vi "scanpic.vi"(8 "error in (no error)":errorcluster, 9 "Size (m)":cluster{"Width":sgl, "Height":sgl}={"Width"=nan, "Height"=nan} caption="Size (m) (NaN=no change)" {"Height" format="%.2p"; "Width" format="%.2p"}, 10 "Application ref in":refnum<vi>, 11 "Center coordinates (m)":cluster{"Xc":sgl, "Yc":sgl}={"Xc"=nan, "Yc"=nan} caption="Center coordinates (m) (NaN=no change)" {"Yc" format="%.2p"; "Xc" format="%.2p"}) -> (0 "Error out":errorcluster, 2 "Application ref out":refnum<vi>, 3 "Data":sgl[][](array[numeric]) format="%#_5p")   [LabVIEW 2020]
uses:
  <userlib>/Nanonis Prog Interface V5/Nanonis Prog Interface.lvlib
panel:
  in  "Channels indexes (0-23) 2":i32[](array[numeric]) caption="Channels indexes (0-23) (Empty=no change)"
  out "Channel name":string
  in  "Channel index (0-23)":u8=14
  out "Signals Names":string[](array[string])
  in  "Pixels":i32 caption="Pixels/line (0=no change)"
  out "Lines":i32
  out "Pixels/line":i32
  out "Channels indexes (0-23)":i32[](array[numeric])
  in  "Serie name":string="ScanMultiBias_"
  in  "Bias increment":sgl
  out "Bias voltage":sgl caption="Current bias voltage"
  out "Scan":u8 caption="Current scan"
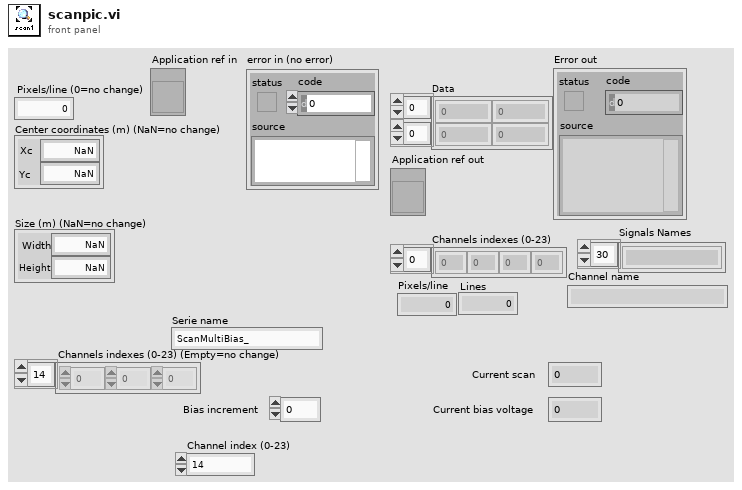
[diagram p1: front panel]
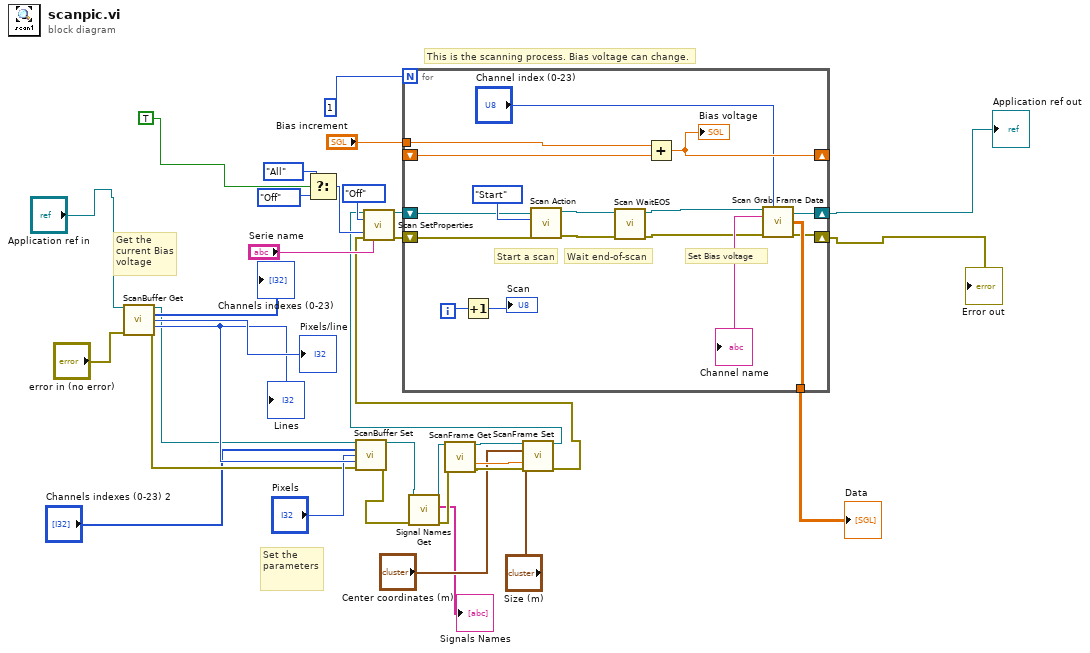
[diagram p0: block diagram]
diagram:
  # "Set the parameters"
  # "This is the scanning process. Bias voltage can change."
  # "Get the current Bias voltage"
  n1 = call <userlib>:"ScanBuffer Get.vi"("Application ref in"="Application ref in", "error in (no error)"="error in (no error)") -> ("Application ref out"=w7:refnum<vi>, "Channels indexes (0-23)"=→"Channels indexes (0-23)":i32[], "Pixels/line"=→"Pixels/line":i32, "Lines"=w25:i32, "error out"=w6:errorcluster)  [unwired: 9 in]
  "Lines" <- w25
  n2 = Select(t=enum16{"No change", "All", "Next", "Off"}."All" ("Auto save"), s=TRUE, f=enum16{"No change", "All", "Next", "Off"}."Off" ("Auto save")) -> (s? t:f=w28:enum16{"No change", "All", "Next", "Off"})
  n3 = call <userlib>:"ScanBuffer Set.vi"("Application ref in"=w7, "Channels indexes (0-23)"="Channels indexes (0-23) 2", "Pixels"="Pixels", "Lines"=w25, "error in (no error)"=w6) -> ("Application ref out"=w13:refnum<vi>, "error out"=w12:errorcluster)  [unwired: 9 in]
  n4 = call <userlib>:"Signal Names Get.vi"("error in (no error)"=w12, "Application ref in"=w13) -> ("error out"=w10:errorcluster, "Signals Names"=→"Signals Names":string[], "Application ref out"=w11:refnum<vi>)  [unwired: 5 in]
  n5 = call <userlib>:"ScanFrame Get.vi"("Application ref in"=w11, "error in (no error)"=w10) -> ("Application ref out"=w23:refnum<vi>, "Angle (deg)"=w22:sgl, "error out"=w21:errorcluster)  [unwired: 9 in, 2 out]
  n6 = call <userlib>:"ScanFrame Set.vi"("Application ref in"=w23, "Center coordinates (m)"="Center coordinates (m)", "Size (m)"="Size (m)", "Angle (deg)"=w22, "error in (no error)"=w21) -> ("Application ref out"=w3:refnum<vi>, "error out"=w4:errorcluster)  [unwired: 9 in]
  n7 = call <userlib>:"Scan SetProperties.vi"("Application ref in"=w3, "Continuous scan"=enum16{"No change", "On", "Off"}."Off", "Auto save"=w28, "Error in (no error)"=w4, "Serie name"="Serie name") -> ("Application ref out"=w27:refnum<vi>, "Error out"=w33:errorcluster)  [unwired: 9 in]
  n8 = for {
    N: 1 -> [_]
    tunnel: "Bias increment" -> [w51]
    shift-right: [w37] -> w1
    shift-left: w33 -> [w39]
    shift-right: [w47] -> _
    shift-left: _ -> [w48]
    shift-right: [w38] -> w2
    shift-left: w27 -> [w40]
    tunnel: [w45] -> w18
    i -> [w50]
    # "Set Bias voltage"
    # "Wait end-of-scan"
    # "Start a scan"
    n9 = Increment(x=w50) -> (x+1=→"Scan":i32)
    n10 = call <userlib>:"Scan Action.vi"("error in (no error)"=w39, "Scan action (Start)"=enum16{"Start", "Stop", "Pause", "Resume"}."Start" ("Scan action"), "Application ref in"=w40) -> ("error out"=w41:errorcluster, "Application ref out"=w42:refnum<vi>)  [unwired: 6 in]
    n11 = call <userlib>:"Scan WaitEOS.vi"("error in (no error)"=w41, "Application ref in"=w42) -> ("error out"=w35:errorcluster, "Application ref out"=w36:refnum<vi>)  [unwired: 5 in, 2 out]
    n12 = Add(x=w51, y=w48) -> (x+y=w47:sgl)
    "Bias voltage" <- w47
    n13 = call <userlib>:"Scan Grab Frame Data.vi"("Application ref in"=w36, "Channel index (0-23)"="Channel index (0-23)", "error in (no error)"=w35) -> ("Application ref out"=w38:refnum<vi>, "Channel name"=→"Channel name":string, "Scan frame data"=w45:sgl[][], "error out"=w37:errorcluster)  [unwired: 8 in, 1 out]
  }
  "Data" <- w18
  "Application ref out" <- w2
  "Error out" <- w1
